vi "PXDAC4800_SessionStreamCreateXD48.vi"(0 "Handle":u32, 5 "StreamingParms":T1) -> (4 "StreamSessionHandle":u32, 6 "Status":i32)   [LabVIEW 2016]
uses:
  PXDAC4800.dll
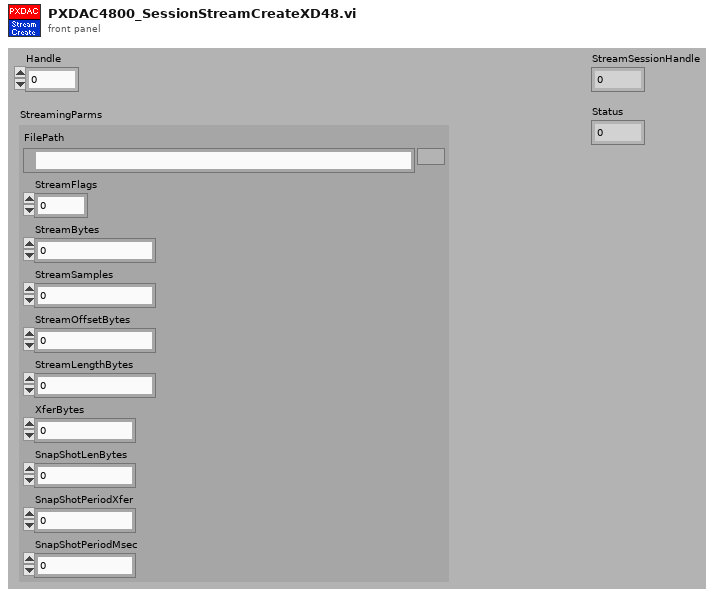
[diagram p1: front panel]
types:
  T1 = cluster{"FilePath":path, "StreamFlags":i32, "StreamBytes":dbl, "StreamSamples":dbl, "StreamOffsetBytes":dbl, "StreamLengthBytes":dbl, "XferBytes":u32, "SnapShotLenBytes":u32, "SnapShotPeriodMsec":u32, "SnapShotPeriodXfer":u32}
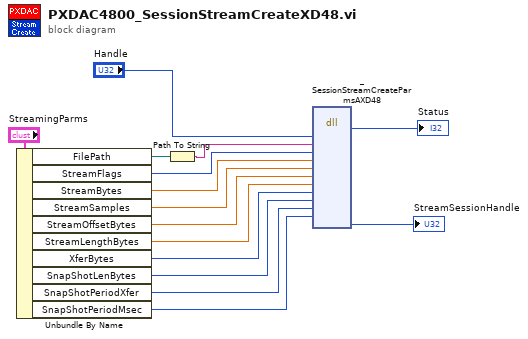
[diagram p0: block diagram]
diagram:
  n1 = Unbundle By Name("StreamingParms") -> ("FilePath"=w11:path, "StreamFlags"=w9:i32, "StreamBytes"=w8:dbl, "StreamSamples"=w7:dbl, "StreamOffsetBytes"=w6:dbl, "StreamLengthBytes"=w5:dbl, "XferBytes"=w4:u32, "SnapShotLenBytes"=w3:u32, "SnapShotPeriodXfer"=w2:u32, "SnapShotPeriodMsec"=w1:u32)
  n2 = Path To String(path=w11) -> (string=w10:string)
  n3 = dll-call lib="PXDAC4800.dll" fn="_SessionStreamCreateParmsAXD48"("Handle"="Handle", "Path"=w10, "StreamFlags"=w9, "StreamBytes"=w8, "StreamSamples"=w7, "StreamOffset"=w6, "StreamLength"=w5, "XferBytes"=w4, "SsLenBytes"=w3, "SsPeriodXfer"=w2, "SsPeriodMs"=w1) -> (→"Status":i32, "Handle"=→"StreamSessionHandle":u32)  [unwired: 15 in, 2 out]
